vi "Initialize.vi"(0 "VisaCluster":T1, 1 "Serial Configuration":T2={"Baud Rate"=19200, "Parity"=0, "Data Bits"=8, "Stop Bits"=10, "Flow Control"=0} {"Flow Control" items=["None", "XON/XOFF", "RTS/CTS", "XON/XOFF & RTS/CTS", "DTR/DSR", "XON/XOFF & DTR/DSR"]; "Stop Bits" items=["1.0"=10, "1.5"=15, "2.0"=20]; "Data Bits" items=["7"=7, "8"=8]; "Parity" items=["None", "Odd", "Even", "Mark", "Space"]; "Baud Rate" items=["300"=300, "600"=600, "1200"=1200, "2400"=2400, "4800"=4800, "9600"=9600, "19200"=19200]}, 11 "error in (no error)":errorcluster) -> (4 "VisaCluster":T1, 15 "error out":errorcluster)   [LabVIEW 2014, in "FH 55.lvlib"]
doc: "Establishes communication with the instrument and optionally performs an instrument identification query and/or an instrument reset. Call this VI before calling other instrument driver VIs for this instrument. Generally, you need to call the Initialize VI only once at the beginning of an application."
uses:
  FH 55.lvlib
  TypeDef/VisaCluster.ctl
panel:
  out "Answer":string
  # "(c) 2010 <Marko Rotkvic>.  ALL RIGHTS RESERVED."
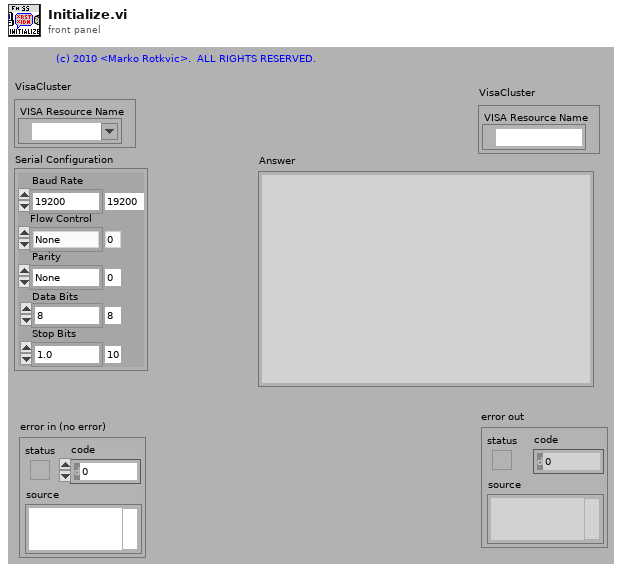
[diagram p1: front panel]
types:
  T1 = typedef "FH 55.lvlib/VisaCluster.ctl" = cluster{"VISA Resource Name":refnum<visa-resource-name>}
  T2 = cluster{"Baud Rate":u32, "Parity":u16, "Data Bits":u16, "Stop Bits":u16, "Flow Control":u16}
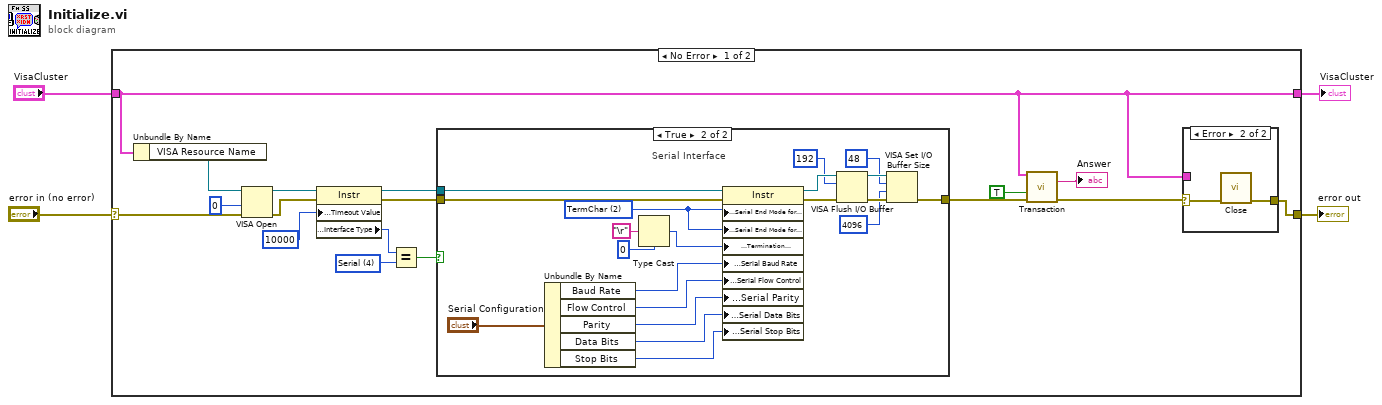
[diagram p0: block diagram]
diagram:
  n1 = case shown="No Error" "error in (no error)" {
    selector: "error in (no error)" -> [w14 w46]
    tunnel: "VisaCluster" -> [w7 w47]
    tunnel: [w7 w47] -> w1
    tunnel: [w12 w46] -> w2
    frame No Error {
      w16 = u16 4 items=["GPIB"=1, "VXI"=2, "GPIB-VXI"=3, "Serial"=4, "PXI"=5, "TCPIP"=6, "USB"=7] ("Interface Information:Interface Type")
      n2 = Unbundle By Name(w7) -> ("VISA Resource Name"=w13:refnum<visa-resource-name>)
      n3 = VISA Open(access mode=u32 0, error in (no error)=w14, VISA resource name=w13) -> (VISA resource name=w10:refnum<visa-resource-name>, error out=w11:errorcluster)  [unwired: 2 in]
      n4 = property class="Instr"(reference=w10, error in=w11, "General Settings:Timeout Value"=u32 10000) -> (reference out=w19:refnum<visa-resource-name>, error out=w18:errorcluster, "Interface Information:Interface Type"=w21:u16)
      n5 = Equal?(x=w21, y=w16) -> (x = y?=w17:bool)
      n6 = case shown="True" w17 {
        tunnel: [w25 w40] -> w9
        tunnel: w19 -> [_ w44]
        tunnel: w18 -> [w25 w45]
        frame False {
          # "GPIB, TCP/IP, and USB Interface"
        }
        frame True {
          w34 = u16 2 items=["None", "LastBit", "TermChar"] ("Serial Settings:Serial End Mode for Reads")
          # "Serial Interface"
          n7 = Unbundle By Name("Serial Configuration") -> ("Baud Rate"=w32:u32, "Flow Control"=w28:u16, "Parity"=w30:u16, "Data Bits"=w31:u16, "Stop Bits"=w27:u16)
          n8 = Type Cast(type=u8 0, x="\r") -> (*(type *) &x=w33:u8)
          n9 = property class="Instr"(reference=w44, error in=w45, "Serial Settings:Serial End Mode for Reads"=w34, "Serial Settings:Serial End Mode for Writes"=w34, "Message Based Settings:Termination Character"=w33, "Serial Settings:Serial Baud Rate"=w32, "Serial Settings:Serial Flow Control"=w28, "Serial Settings:Serial Parity"=w30, "Serial Settings:Serial Data Bits"=w31, "Serial Settings:Serial Stop Bits"=w27) -> (reference out=w39:refnum<visa-resource-name>, error out=w42:errorcluster)
          n10 = VISA Flush I/O Buffer(VISA resource name=w39, mask (16)=u16 192, error in (no error)=w42) -> (VISA resource name out=w43:refnum<visa-resource-name>, error out=w41:errorcluster)
          n11 = VISA Set I/O Buffer Size(VISA resource name=w43, mask (16)=u16 48, size (4096)=u32 4096 ("size (0)"), error in (no error)=w41) -> (error out=w40:errorcluster)  [unwired: 1 out]
        }
      }
      n12 = call "Transaction.vi"("VisaCluster"=w7, "Read Only? (False)"=TRUE ("Read Only? (True)"), "error in (no error)"=w9) -> ("Answer"=→"Answer":string, "error out"=w5:errorcluster)  [unwired: 9 in, 2 out]
      n13 = case shown="Error" w5 {
        selector: w5 -> [w22 w23]
        tunnel: [w22 w24] -> w12
        tunnel: w7 -> [_ _]
        frame No Error {
        }
        frame Error {
          n14 = call "Close.vi"("error in (no error)"=w23) -> ("error out"=w24:errorcluster)  [unwired: 14 in]
        }
      }
    }
    frame Error {
    }
  }
  "error out" <- w2
  "VisaCluster" <- w1
